vi "Load TS DAC Configuration.vi"(8 "error in":errorcluster, 11 "Test Stand in":refnum<class "Generic Test Stand.lvclass">) -> (0 "error out":errorcluster, 1 "Ctrl Interval":dbl, 2 "Trig Resolution":u32, 3 "Test Stand out":refnum<class "Generic Test Stand.lvclass">)   [LabVIEW 2019, in "Generic Test Stand.lvclass"]
uses:
  Generic Test Stand.lvclass
  Generic Test Stand.lvclass/Generic Test Stand.ctl
  DAC/DAC.lvclass
  <vilib>/Utility/config.llb/NI_LVConfig.lvlib
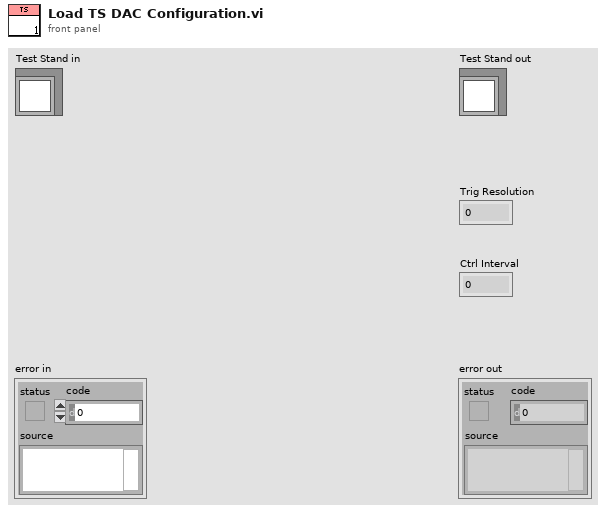
[diagram p1: front panel]
types:
  T1 = typedef "NI_LVConfig.lvlib/Config Data RefNum.ctl" = refnum<k1>
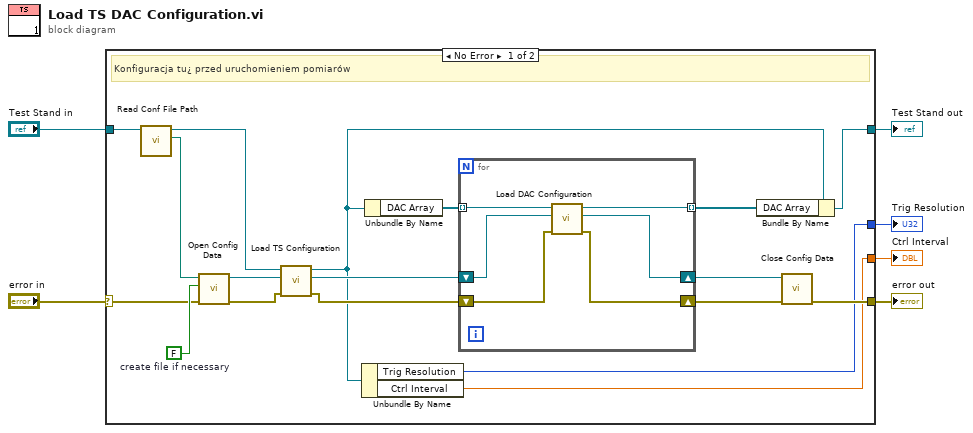
[diagram p0: block diagram]
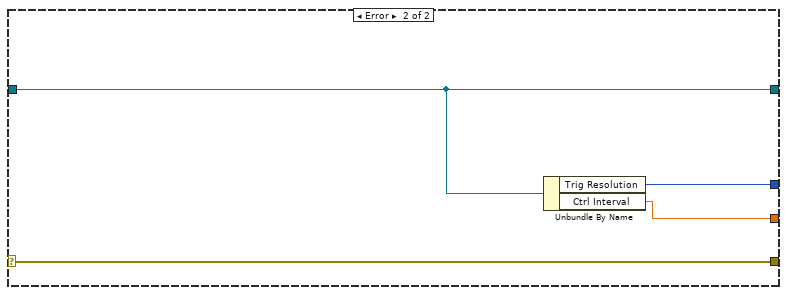
[diagram p2: hidden frame]
diagram:
  n1 = case shown="No Error" "error in" {
    selector: "error in" -> [w8 w34]
    tunnel: "Test Stand in" -> [w16 w33]
    tunnel: [w17 w33] -> w4
    tunnel: [w20 w34] -> w3
    tunnel: [w9 w32] -> w2
    tunnel: [w7 w31] -> w1
    frame No Error {
      w23 = FALSE  # create file if necessary
      # "Konfiguracja tu¿ przed uruchomieniem pomiarów"
      n2 = call "Read Conf File Path.vi"("Generic Test Stand in"=w16) -> ("Conf File Path"=w24:path, "Generic Test Stand out"=w14:refnum<class "Generic Test Stand.lvclass">)  [unwired: 8 in, 1 out]
      n3 = call <vilib>:"Open Config Data.vi"("error in (no error)"=w8, "create file if necessary (T)"=w23, "configuration file path"=w24) -> ("error out"=w13:errorcluster, "refnum"=w15:T1)  [unwired: 6 in, 1 out]
      n4 = call-dynamic "Load TS Configuration.vi"("error in"=w13, "Config File refnum in"=w15, "Generic Test Stand in"=w14) -> ("error out"=w11:errorcluster, "Config File refnum out"=w12:T1, "Generic Test Stand out"=w10:refnum<class "Generic Test Stand.lvclass">)  [unwired: 6 in]
      n5 = Unbundle By Name(w10) -> ("Trig Resolution"=w9:u32, "Ctrl Interval"=w7:dbl)
      n6 = Unbundle By Name(w10) -> ("DAC Array"=w19:refnum<class "DAC.lvclass">[])
      n7 = for {
        tunnel: w19 -> [w29] mode=indexing
        tunnel: [w28] -> w18 mode=indexing
        shift-right: [w25] -> w22
        shift-left: w11 -> [w26]
        shift-right: [w27] -> w21
        shift-left: w12 -> [w30]
        n8 = call-dynamic "Load DAC Configuration.vi"("error in"=w26, "Config File refnum in"=w30, "DAC in"=w29) -> ("error out"=w25:errorcluster, "Config File refnum out"=w27:T1, "DAC out"=w28:refnum<class "DAC.lvclass">)  [unwired: 6 in]
      }
      n9 = Bundle By Name(cluster=w10, "DAC Array"=w18) -> (w17:refnum<class "Generic Test Stand.lvclass">)
      n10 = call <vilib>:"Close Config Data.vi"("error in (no error)"=w22, "refnum"=w21) -> ("error out"=w20:errorcluster)  [unwired: 8 in, 1 out]
    }
    frame Error {
      n11 = Unbundle By Name(w33) -> ("Trig Resolution"=w32:u32, "Ctrl Interval"=w31:dbl)
    }
  }
  "error out" <- w3
  "Test Stand out" <- w4
  "Trig Resolution" <- w2
  "Ctrl Interval" <- w1
